vi "Yoyo_Setup.vi"(11 "Ele_Pos_Yoyo":T1) -> (3 "Ele_Pos_Yoyo":dbl)   [LabVIEW 2014]
uses:
  <vilib>/Rock Robotics/WPI/AnalogChannel/WPI_AnalogChannelDevRef.ctl
  <vilib>/Rock Robotics/SystemInterfaces/Typedef/FPGA_TypedefAnalogModule.ctl
  <vilib>/Rock Robotics/SystemInterfaces/AI/FPGA_AIChannel.ctl
  General_VI/Global Var.vi
panel:
  in  "Ele_Pos_Inch":dbl[](array[numeric])=[8.125, 23.0, 34.5, 46.25, 52.625, 54.3125]
  in  "Ele_Voltage":dbl[](array[numeric])=[0.4748, 1.87, 2.98, 4.1, 4.729, 4.9]
  out "Elev_Map":cluster{"X_Array":dbl[], "Y_Array":dbl[]}(graph)
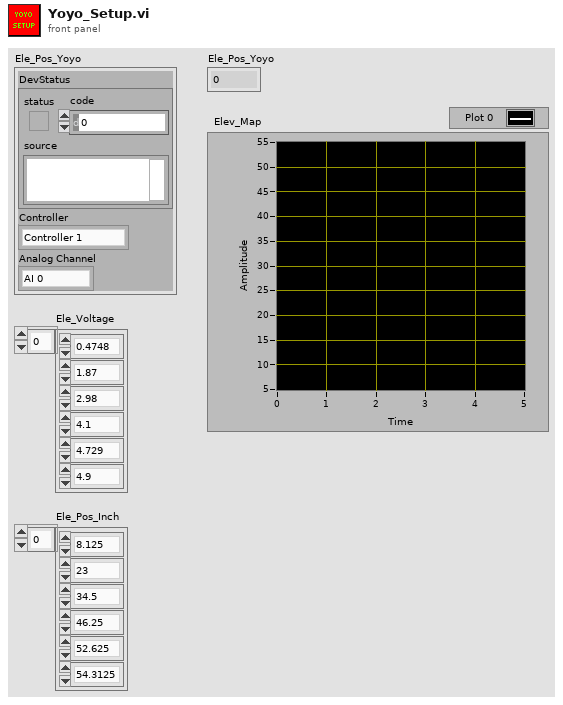
[diagram p1: front panel]
types:
  T1 = typedef "WPI_AnalogChannelDevRef.ctl" = cluster{"DevStatus":errorcluster, "Controller":T2, "Analog Channel":T3}
  T2 = typedef "FPGA_TypedefAnalogModule.ctl" = enum16{"Controller 1"}
  T3 = typedef "FPGA_AIChannel.ctl" = enum8{"AI 0", "AI 1", "AI 2", "AI 3", "AI MXP 0", "AI MXP 1", "AI MXP 2", "AI MXP 3", "Invalid"}
  T4 = cluster{"Ele_Voltage":dbl[], "Ele_Pos_Inch":dbl[]}
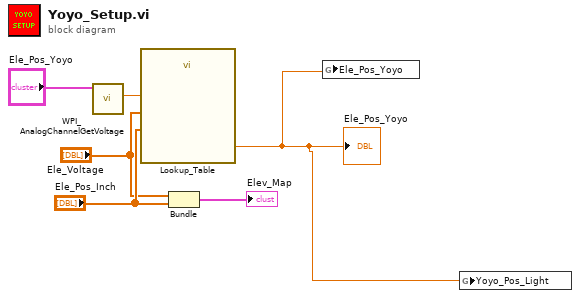
[diagram p0: block diagram]
diagram:
  n1 = call <vilib>:"WPI_AnalogChannelGetVoltage.vi"("AIDeviceRef"="Ele_Pos_Yoyo") -> ("Voltage"=w4:dbl)  [unwired: 8 in, 2 out]
  n2 = call "Lookup_Table.vi"("Y_Array"="Ele_Pos_Inch", "x_in"=w4, "X_Array"="Ele_Voltage") -> ("y_out"=w1:dbl)  [unwired: 6 in]
  "Ele_Pos_Yoyo" <- w1
  n3 = Bundle("Ele_Voltage"="Ele_Voltage", "Ele_Pos_Inch"="Ele_Pos_Inch") -> (→"Elev_Map":T4)  [unwired: 1 in]
  n4 = global write "Global Var.vi" "Ele_Pos_Yoyo"(w1) -> ()
  n5 = global write "Global Var.vi" "Yoyo_Pos_Light"(w1) -> ()
